vi "Execute.vi"(8 "error in":errorcluster, 11 "Ozone Addition Valve in":refnum<class "Ozone Addition Valve.lvclass">) -> (0 "error out":errorcluster, 1 "Next Step?":bool, 2 "MSG":string, 3 "Ozone Addition Valve out":refnum<class "Ozone Addition Valve.lvclass">)   [LabVIEW 2015, in "Ozone Addition Valve.lvclass"]
uses:
  Ozone Addition Valve.lvclass
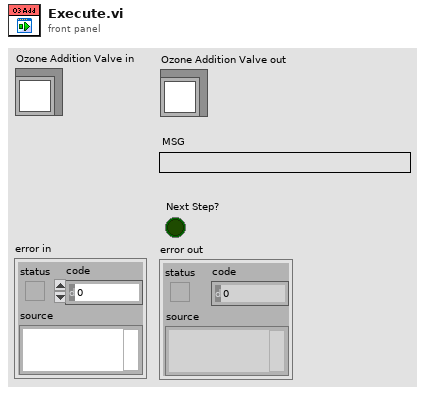
[diagram p1: front panel]
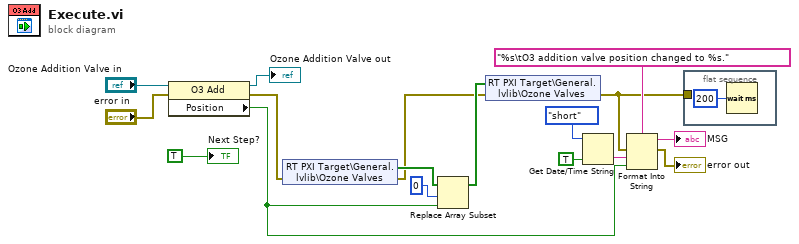
[diagram p0: block diagram]
diagram:
  n1 = property class="O3 Add"(reference="Ozone Addition Valve in", error in="error in") -> (reference out=→"Ozone Addition Valve out":refnum<class "Ozone Addition Valve.lvclass">, error out=w3:errorcluster, "Position"=w5:bool)
  n2 = shared-variable "RT PXI Target\\General.lvlib\\Ozone Valves"(error in=w3) -> (w7:bool[], error out=w2:errorcluster)
  n3 = Replace Array Subset(array=w7, new element=w5, index=0) -> (w4:bool[])
  n4 = shared-variable "RT PXI Target\\General.lvlib\\Ozone Valves"(w4, error in=w2) -> (error out=w1:errorcluster)
  n5 = Get Date/Time String(date format (0)=enum16{"short", "long", "abbreviated"}."short", want seconds? (F)=TRUE) -> (time string=w15:string)  [unwired: 1 in, 1 out]
  n6 = Format Into String(format string="%s\tO3 addition valve position changed to %s.", error in=w1, w15, w5) -> (resulting string=→"MSG":string, error out=→"error out":errorcluster)  [unwired: 1 in]
  n7 = flat-sequence {
    tunnel: w1 -> [_]
    frame #0 {
      n8 = Wait (ms)(milliseconds to wait=u32 200) -> ()  [unwired: 1 out]
    }
  }
  "Next Step?" <- TRUE ("Next Step?")
